vi "host.vi"() -> ()   [LabVIEW 2020]
uses:
  <vilib>/Analysis/baseanly.llb/Real A x B.vi
  <vilib>/Analysis/Matrix/Numeric/Conversions/Matrix To Array - RM.vi
  <vilib>/FPGAPlugInAG/cRIO-9035/niLvFpga_Open_cRIO-9035.vi
  <vilib>/rvi/interface/common/dynamic/niFpgaDynamicAddResources.vi
  <vilib>/Utility/error.llb/Error Cluster From Error Code.vi
  <vilib>/rvi/errors/niLvFpgaAdjustHostInterfaceError.vi
  <vilib>/FPGAPlugInAG/Dynamic/niLvFpga_Run_Dynamic.vi
  <vilib>/FPGAPlugInAG/Dynamic/niLvFpga_Close_Dynamic.vi
  <vilib>/rvi/interface/nirviOpenFPGA/nirviOpenFPGA.xnode
  FPGA Bitfiles/checkpolymorphic_FPGATarget_target_+xb45D36SCA.lvbitx
  target.vi
  <vilib>/rvi/interface/nirviMethod/nirviMethod.xnode
  <vilib>/rvi/interface/nirviReadWriteControl/nirviReadWriteControl.xnode
  <vilib>/rvi/interface/nirviCloseFPGA/nirviCloseFPGA.xnode
  <vilib>/FPGAPlugInAG/Dynamic/niLvFpga_WriteFifo_Dynamic.vi
  <vilib>/rvi/errors/niLvFpgaMergeErrorWithErrorCode.vi
  <vilib>/Analysis/NI_AALBase.lvlib
  <vilib>/Analysis/Matrix/NI_Matrix.lvlib
  NiFpgaLv.dll
  <vilib>/rvi/interface/Simulation/niFpgaSimulationCallBeginRW.vi
  <vilib>/FPGAPlugInAG/Dynamic/niLvFpga_ReadFifo_Dynamic.vi
panel:
  out "x*y":dbl
  out "ticks":u32
  out "elements in B":i32
  out "elements in A":i32
  out "sum of error":dbl
  out "C - FPGA code":sgl[][](array[numeric])
  out "elements in C":i32
  out "C - Real":dbl[][](array[numeric])
  out "B":sgl[][](array[numeric])
  out "A":sgl[][](array[numeric])
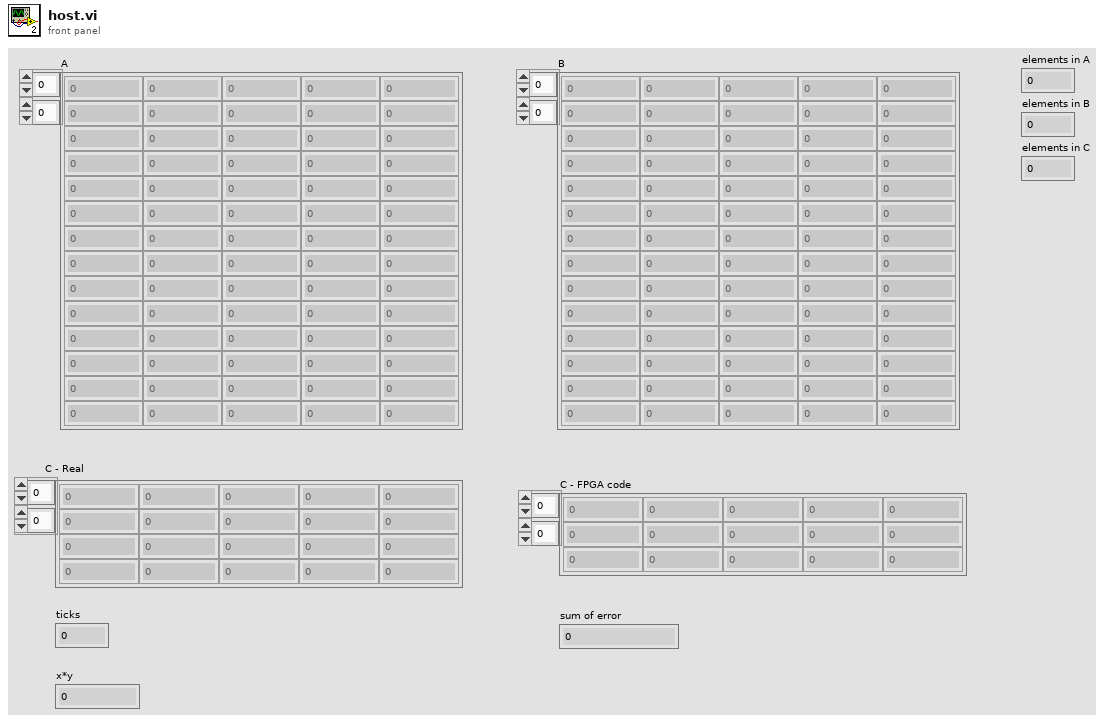
[diagram p1: front panel]
types:
  T1 = typedef "NI_Matrix.lvlib/RealMatrix.ctl" = dbl[][]
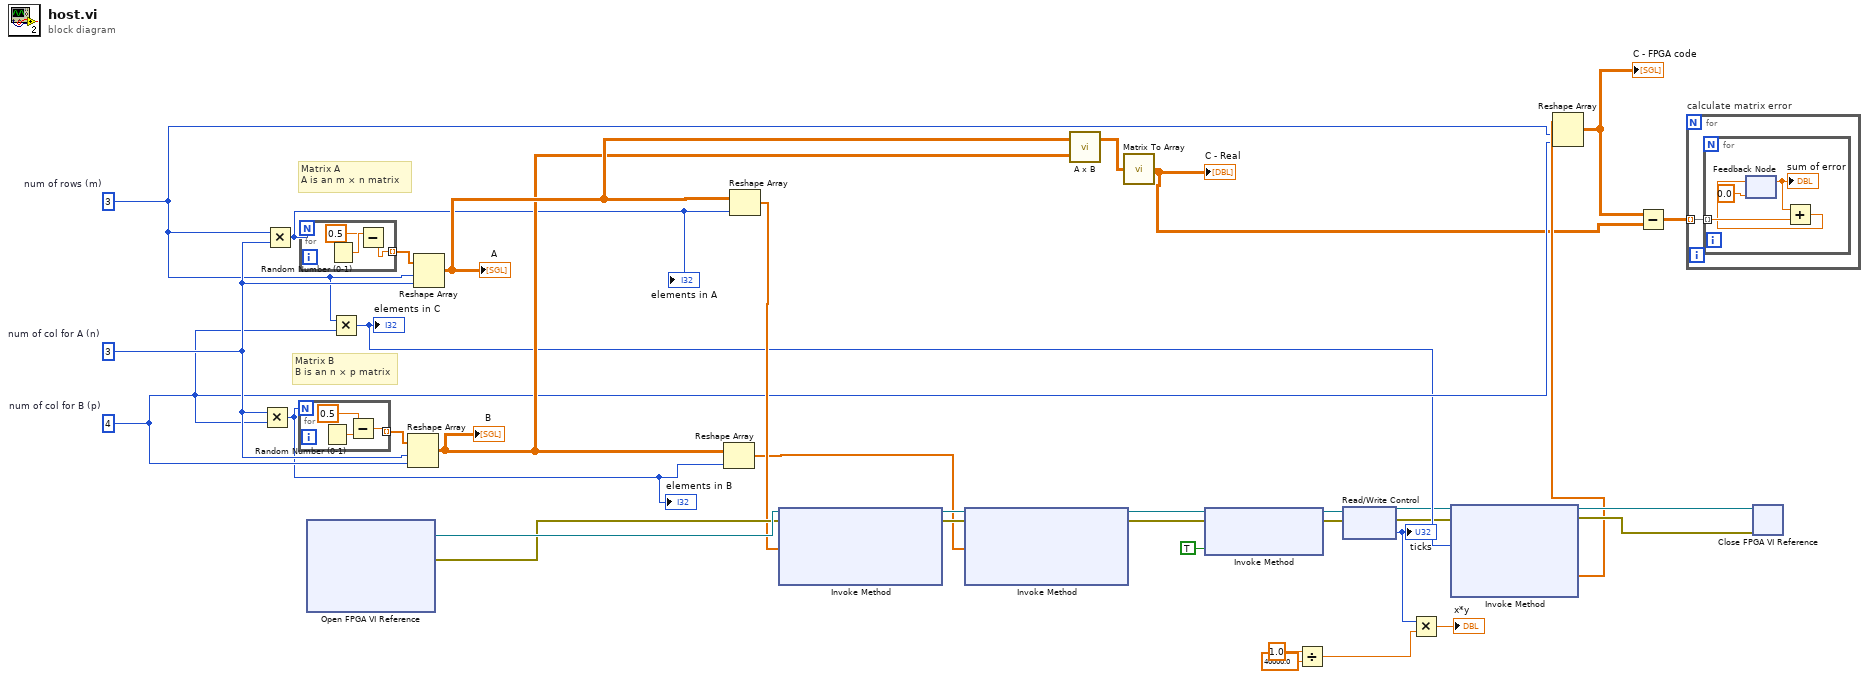
[diagram p0: block diagram]
diagram:
  w13 = 4  # num of col for B (p)
  w20 = 3  # num of col for A (n)
  w14 = 3  # num of rows (m)
  # "Matrix B\nB is an n × p matrix"
  # "Matrix A\nA is an m × n matrix"
  n1 = Multiply(x=w20, y=w13) -> (x*y=w10:i32)
  "elements in B" <- w10
  n2 = Multiply(x=w14, y=w20) -> (x*y=w21:i32)
  "elements in A" <- w21
  n3 = for {
    N: w10 -> [_]
    tunnel: [w37] -> w25 mode=indexing
    n4 = Random Number (0-1)() -> (number: 0 to 1=w38:dbl)
    n5 = Subtract(x=w38, y=sgl 0.5) -> (x-y=w37:sgl)
  }
  n6 = for {
    N: w21 -> [_]
    tunnel: [w40] -> w26 mode=indexing
    n7 = Random Number (0-1)() -> (number: 0 to 1=w41:dbl)
    n8 = Subtract(x=w41, y=sgl 0.5) -> (x-y=w40:sgl)
  }
  n9 = xnode "Open FPGA VI Reference"() -> ("FPGA VI Reference Out"=w34:refnum<k20>, "error out"=w33:errorcluster)  [unwired: 2 in]
  n10 = Multiply(x=w14, y=w13) -> (x*y=w11:i32)
  "elements in C" <- w11
  n11 = Reshape Array(w25, w20, w13) -> (w23:sgl[][])
  "B" <- w23
  n12 = Reshape Array(w26, w14, w20) -> (w24:sgl[][])
  "A" <- w24
  n13 = Reshape Array(w23, w10) -> (w18:sgl[])
  n14 = Reshape Array(w24, w21) -> (w19:sgl[])
  n15 = xnode "Invoke Method"("FPGA VI Reference In"=w34, "error in"=w33, "Data"=w19) -> ("FPGA VI Reference Out"=w30:refnum<k20>, "error out"=w29:errorcluster)  [unwired: 1 in, 1 out]
  n16 = xnode "Invoke Method"("FPGA VI Reference In"=w30, "error in"=w29, "Data"=w18) -> ("FPGA VI Reference Out"=w28:refnum<k20>, "error out"=w27:errorcluster)  [unwired: 1 in, 1 out]
  n17 = call-poly <vilib>:"A x B.vi"("B"=w23, "A"=w24) -> ("A x B"=w22:T1)  [unwired: 1 out]
  n18 = call-poly <vilib>:"Matrix To Array.vi"("Real Matrix"=w22) -> ("Real 2D Array"=w12:dbl[][])
  "C - Real" <- w12
  n19 = xnode "Invoke Method"("FPGA VI Reference In"=w28, "error in"=w27, "Wait Until Done (F)"=TRUE) -> ("FPGA VI Reference Out"=w9:refnum<k20>, "error out"=w8:errorcluster)
  n20 = Divide(x=1.0, y=40000.0) -> (x/y=w2:dbl)
  n21 = xnode "Read/Write Control"("FPGA VI Reference In"=w9, "error in"=w8) -> ("FPGA VI Reference Out"=w7:refnum<k20>, "error out"=w6:errorcluster, "ticks"=w5:u32)
  "ticks" <- w5
  n22 = Multiply(x=w5, y=w2) -> (x*y=→"x*y":dbl)
  n23 = xnode "Invoke Method"("FPGA VI Reference In"=w7, "error in"=w6, "Number of Elements"=w11) -> ("FPGA VI Reference Out"=w32:refnum<k20>, "error out"=w31:errorcluster, "Data"=w15:sgl[])  [unwired: 1 in, 1 out]
  n24 = Reshape Array(w15, w14, w13) -> (w17:sgl[][])
  "C - FPGA code" <- w17
  n25 = Subtract(x=w17, y=w12) -> (x-y=w16:dbl[][])
  n26 = for "calculate matrix error" {
    tunnel: w16 -> [w42] mode=indexing
    n27 = for {
      tunnel: w42 -> [w46] mode=indexing
      n28 = feedback #1(0.0) -> (w44:dbl)
      "sum of error" <- w44
      n29 = Add(x=w44, y=w46) -> (x+y=w45:dbl)
      n30 = feedback-in #1(w45) -> ()
    }
  }
  n31 = xnode "Close FPGA VI Reference"("FPGA VI Reference In"=w32, "error in"=w31) -> ()  [unwired: 1 out]
